vi "upper left to center.vi"(10 "target size":cluster{"sx":i32, "sy":i32}, 11 "ponto in":cluster{"X":dbl, "Y":dbl}[](array[cluster])) -> (3 "ponto out":cluster{"X":dbl, "Y":dbl}[](array[cluster]))   [LabVIEW 2016]
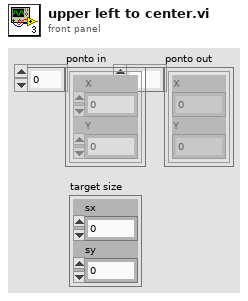
[diagram p1: front panel]
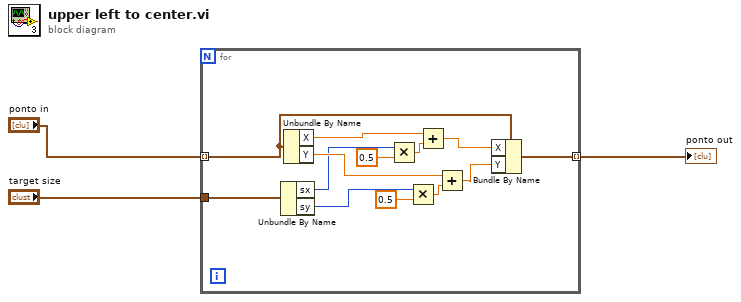
[diagram p0: block diagram]
diagram:
  n1 = for {
    tunnel: "target size" -> [w4]
    tunnel: "ponto in" -> [w15] mode=indexing
    tunnel: [w16] -> w3 mode=indexing
    n2 = Unbundle By Name(w4) -> ("sx"=w7:i32, "sy"=w14:i32)
    n3 = Unbundle By Name(w15) -> ("X"=w5:dbl, "Y"=w13:dbl)
    n4 = Multiply(x=w7, y=sgl 0.5) -> (x*y=w6:sgl)
    n5 = Multiply(x=w14, y=sgl 0.5) -> (x*y=w10:sgl)
    n6 = Add(x=w5, y=w6) -> (x+y=w9:dbl)
    n7 = Add(x=w13, y=w10) -> (x+y=w12:dbl)
    n8 = Bundle By Name(cluster=w15, "X"=w9, "Y"=w12) -> (w16:cluster{"X":dbl, "Y":dbl})
  }
  "ponto out" <- w3
